vi "SpecAn Fetch AMPM.vi"(0 "RFmx Handle In":refnum<k21>, 1 "Selector String":string, 11 "error in (no error)":errorcluster) -> (4 "RFmx Handle Out":refnum<k21>, 6 "AMPM Results":T1 {"AM to PM Residual (deg)" format="%.2f"; "AM to AM Residual (dB)" format="%.2f"; "Mean RMS EVM (%)" format="%.2f"; "1 dB Compression Point (dBm)" format="%.2f"; "Mean Linear Gain (dB)" format="%.2f"}, 15 "error out":errorcluster)   [LabVIEW 2019, in "RFmxSpecAn.lvlib"]
doc: "Fetches common results from the AMPM measurement."
uses:
  RFmxSpecAn.lvlib
  Typedefs/SpecAn AMPM Results.ctl
  <vilib>/RFmx/SpecAn/mx/RFmxSpecAn.llb/RFmxSpecAn AMPM Fetch DUT Characteristics.vi
  <vilib>/RFmx/SpecAn/mx/RFmxSpecAn.llb/RFmxSpecAn AMPM Fetch Curve Fit Residual.vi
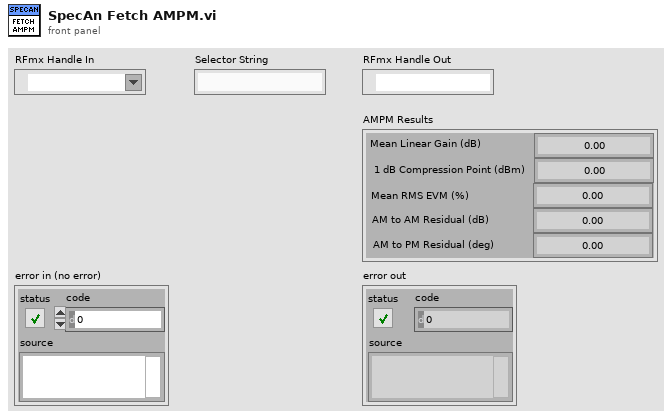
[diagram p1: front panel]
types:
  T1 = typedef "RFmxSpecAn.lvlib/SpecAn AMPM Results.ctl" = cluster{"Mean Linear Gain (dB)":dbl, "1 dB Compression Point (dBm)":dbl, "Mean RMS EVM (%)":dbl, "AM to AM Residual (dB)":dbl, "AM to PM Residual (deg)":dbl}
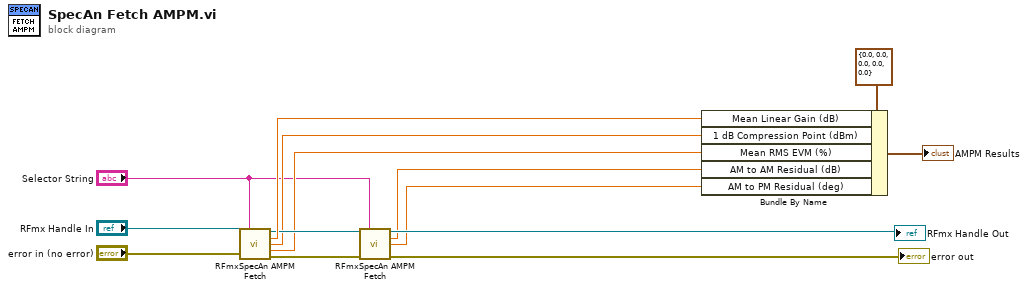
[diagram p0: block diagram]
diagram:
  n1 = call-poly <vilib>:"RFmxSpecAn AMPM Fetch.vi"("Instrument Handle In"="RFmx Handle In", "Selector String"="Selector String", "error in (no error)"="error in (no error)") -> ("Instrument Handle Out"=w9:refnum<k21>, "Mean Linear Gain (dB)"=w12:dbl, "1 dB Compression Point (dBm)"=w7:dbl, "Mean RMS EVM (%)"=w6:dbl, "error out"=w14:errorcluster)  [unwired: 8 in]
  n2 = call-poly <vilib>:"RFmxSpecAn AMPM Fetch.vi"("Instrument Handle In"=w9, "Selector String"="Selector String", "error in (no error)"=w14) -> ("Instrument Handle Out"=→"RFmx Handle Out":refnum<k21>, "AM to AM Residual (dB)"=w5:dbl, "AM to PM Residual (deg)"=w4:dbl, "error out"=→"error out":errorcluster)  [unwired: 9 in]
  n3 = Bundle By Name(cluster=T1 {"Mean Linear Gain (dB)"=0.0, "1 dB Compression Point (dBm)"=0.0, "Mean RMS EVM (%)"=0.0, "AM to AM Residual (dB)"=0.0, "AM to PM Residual (deg)"=0.0} ("AMPM Results"), "Mean Linear Gain (dB)"=w12, "1 dB Compression Point (dBm)"=w7, "Mean RMS EVM (%)"=w6, "AM to AM Residual (dB)"=w5, "AM to PM Residual (deg)"=w4) -> (→"AMPM Results":T1)
